vi "Test Get Plugin Parameter.vi"(8 "error in (no error)":errorcluster, 11 "Configuration Manager Test in":refnum<class "Configuration Manager Test.lvclass">) -> (0 "error out":errorcluster, 3 "Configuration Manager Test out":refnum<class "Configuration Manager Test.lvclass">)   [LabVIEW 2020, in "Configuration Manager Test.lvclass"]
uses:
  Configuration Manager Test.lvclass
  Configuration Manager Test.lvclass/Configuration Manager Test.ctl
  source/User Interface/Configuration Manager/Configuration Manager.lvclass
  da4b3e93-04f0-485b-8eef-eaf6a6b0a3f6.vi
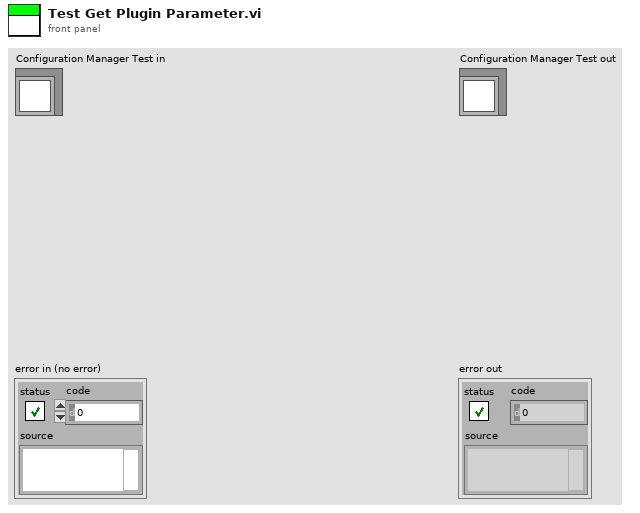
[diagram p1: front panel]
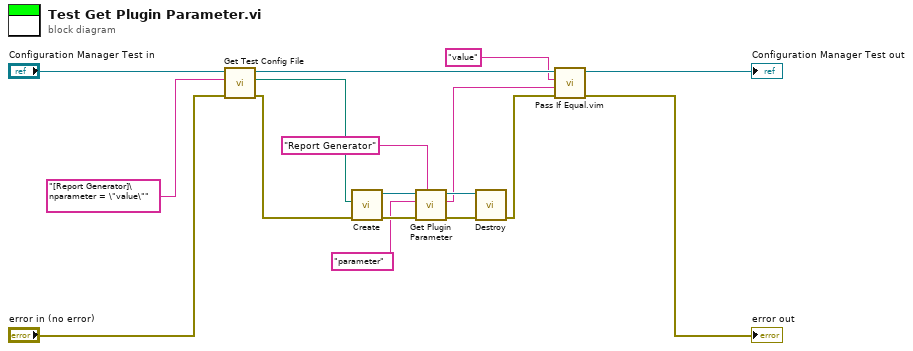
[diagram p0: block diagram]
diagram:
  n1 = call "Get Test Config File.vi"("error in (no error)"="error in (no error)", "File Content"="[Report Generator]\nparameter = \"value\"", "Configuration Manager Test in"="Configuration Manager Test in") -> ("error out"=w10:errorcluster, "File Path"=w5:path, "Configuration Manager Test out"=w7:refnum<class "Configuration Manager Test.lvclass">)  [unwired: 6 in]
  n2 = call "Create.vi"("error in (no error)"=w10, "configuration file path"=w5) -> ("error out"=w13:errorcluster, "Configuration Manager out"=w14:refnum<class "Configuration Manager.lvclass">)  [unwired: 8 in]
  n3 = call "Get Plugin Parameter.vi"("Plugin"="Report Generator", "error in (no error)"=w13, "Name"="parameter", "Configuration Manager in"=w14) -> ("error out"=w11:errorcluster, "Value"=w3:string, "Configuration Manager out"=w12:refnum<class "Configuration Manager.lvclass">)  [unwired: 5 in]
  n4 = call "Destroy.vi"("error in (no error)"=w11, "Configuration Manager In"=w12) -> ("error out"=w9:errorcluster)  [unwired: 9 in]
  n5 = call "Pass If Equal.vim"("error in (no error)"=w9, "Actual"=w3, "Expected"="value" ("Report Path"), "LUnit Test Case In"=w7) -> ("error out"=→"error out":errorcluster, "LUnit Test Case Out"=→"Configuration Manager Test out":refnum<class "Configuration Manager Test.lvclass">)  [unwired: 6 in]
